vi "Project Manager.vi"() -> ()   [LabVIEW 2012]
doc: "This VI performs some project management operations on source trees. In particular, it is can be used to load VIs that are no subVI of the application such as instantiation templates, dynamically loaded VIs, test VIs and so on. By doing so, changes to subVIs or typedefs used throughout the source tree can be applied everywhere, evaluated (any VIs with broken arrows?), and reverted or saved as they are being made instead of waiting for any side effects to show the next time the using VIs in the source tree are loaded.\n\nTo deploy this VI, simply place it and its state typedef in the root directory of your projects VI source tree. To ease this migration, it is designed to not make use of any non-standard subVIs. When run, it will automatically list the VIs by recursing into the lower subdirectories. Thus, the collection of VIs being managed can be changed by moving the VI to a different source tree or by moving VIs into or outside the source tree."
uses:
  t_Project Manager States.ctl
panel:
  in  "exclude":string="^.*\\.ctt?$"
  in  "unload templates":bool
  in  "unload all":bool
  in  "include":string="^.*\\.[cv][ti][lt]?$"
  in  "directory/llb regexp":string
  in  "open selected":bool
  in  "reinitialize":bool
  in  "load all":bool
  in  "file list":i32[](listbox)
  in  "stop":bool
  in  "load selected":bool
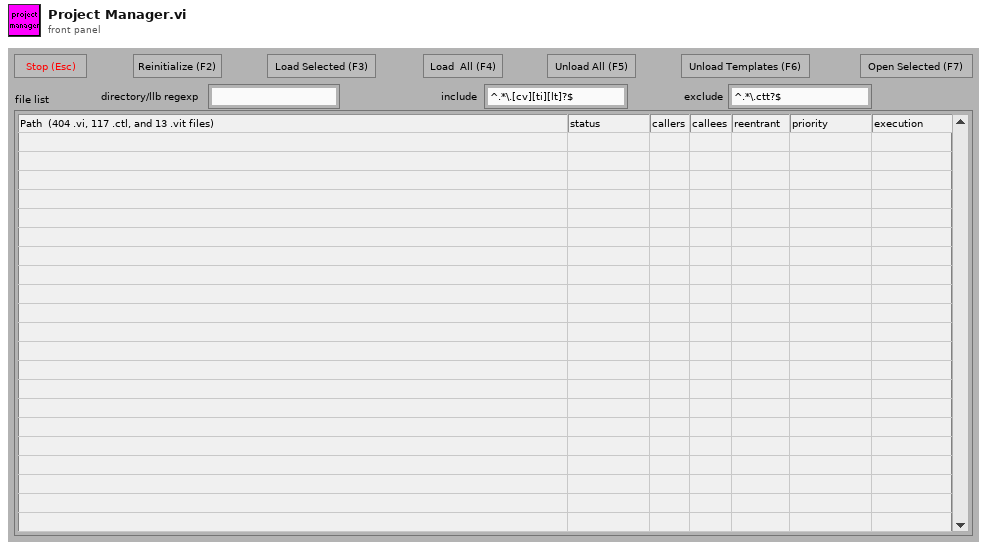
[diagram p1: front panel]
types:
  T1 = typedef "t_Project Manager States.ctl" = enum16{"empty queue", "adjust size", "load", "ld open", "ld calls", "ld system&exec", "unload", "unload templates", "open selected", "update stats", "ablement", "initialize", "cleanup", "stop"}
  T2 = enum32{"Bad", "Idle", "Run top level", "Running"}
  T3 = typedef "eventvkey.ctl" = enum16{"ASCII", "Enter", "Return", "Shift", "Ctrl", "Alt", "Cmd", "Opt", "Caps", "NumLock", "Clear", "Break", "Up", "Down", "Left", "Right", "Insert", "Delete", "Home", "End", "PageUp", "PageDown", "Escape", "Help", "Pause", "ScrollLock", "F1", "F2", "F3", "F4", "F5", "F6", "F7", "F8", "F9", "F10", "F11", "F12", "F13", "F14", "F15", "F16", "F17", "F18", "F19", "F20", "F21", "F22", "F23", "F24", "Play", "VolumeUp", "VolumeDown", "Mute", "Two Byte Char"}
  T4 = enum32{"invalid priority", "background priority", "normal priority", "above normal priority", "high priority", "time critical priority", "subroutine"}
  T5 = enum32{"invalid execution system", "user interface", "standard", "instrument i/o", "data acquisition", "other 1", "other 2", "same as caller"}
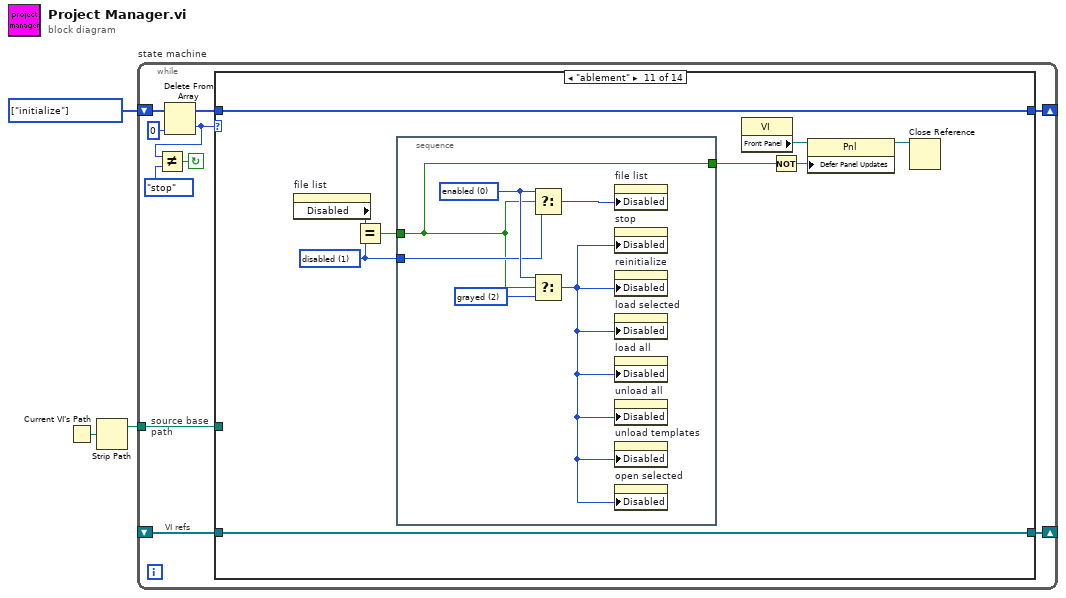
[diagram p0: block diagram]
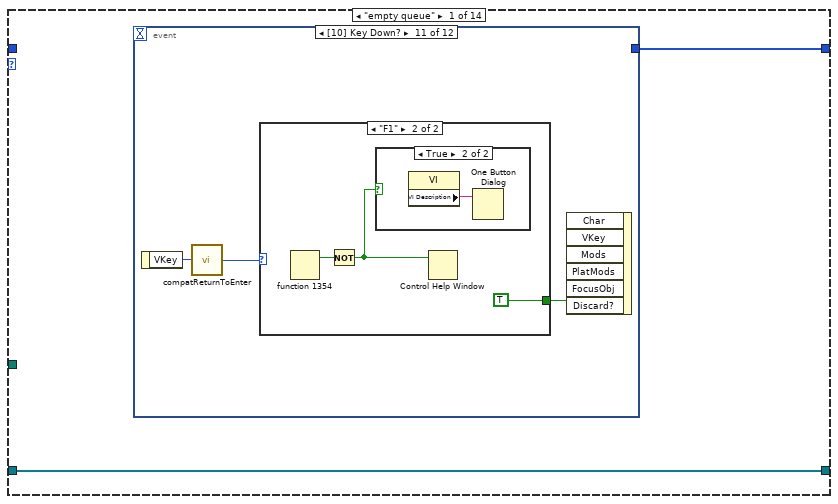
[diagram p2: hidden frame]
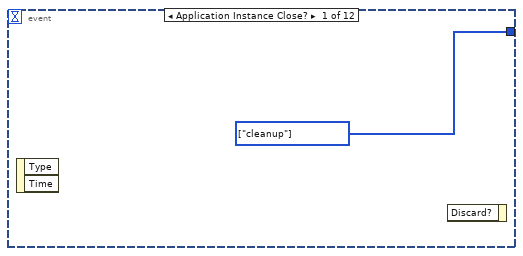
[diagram p3: hidden frame]
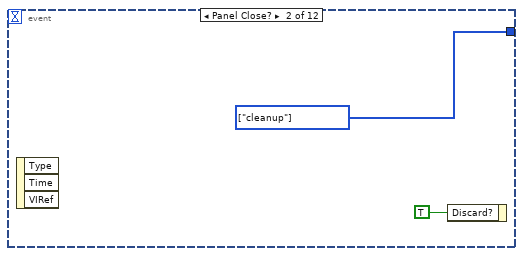
[diagram p4: hidden frame]
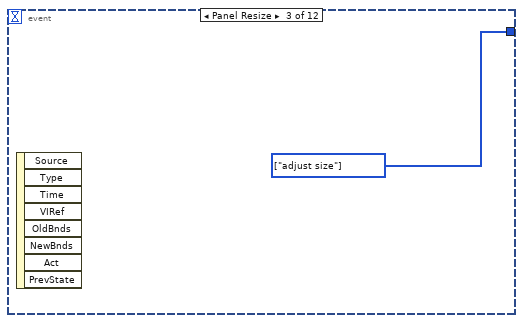
[diagram p5: hidden frame]
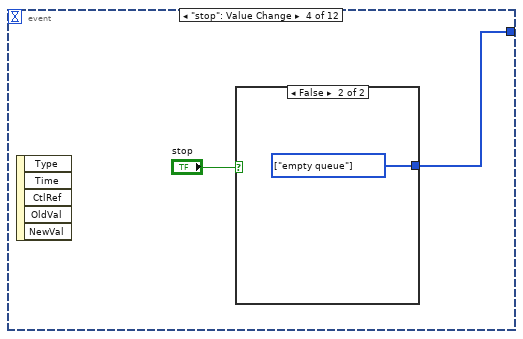
[diagram p6: hidden frame]
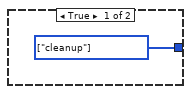
[diagram p7: hidden frame]
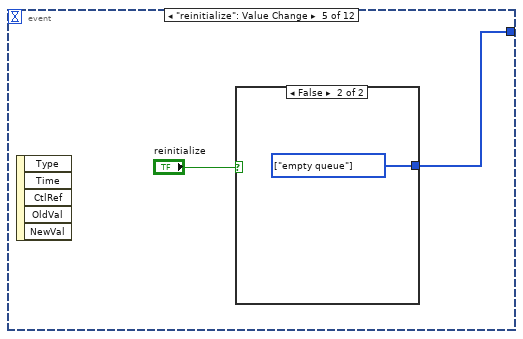
[diagram p8: hidden frame]
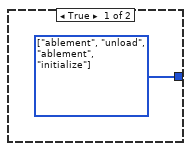
[diagram p9: hidden frame]
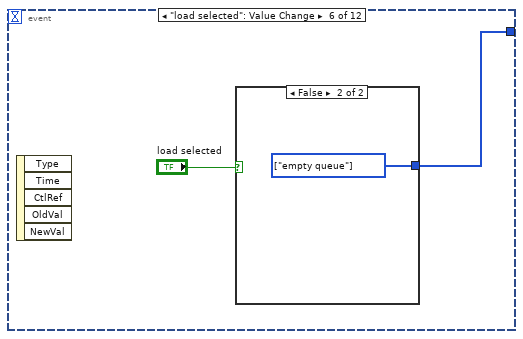
[diagram p10: hidden frame]
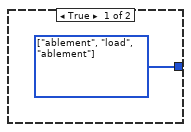
[diagram p11: hidden frame]
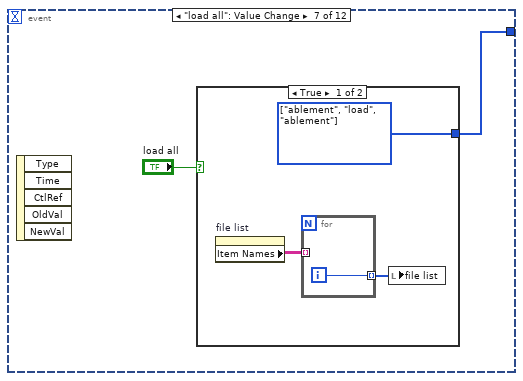
[diagram p12: hidden frame]
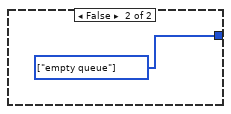
[diagram p13: hidden frame]
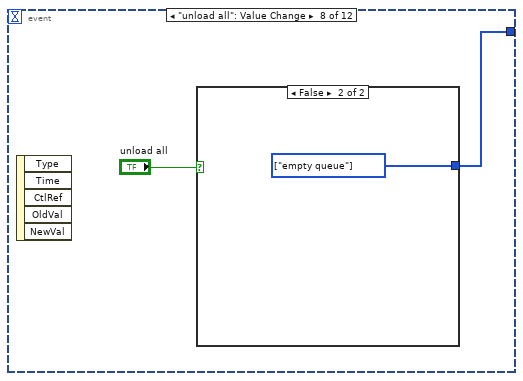
[diagram p14: hidden frame]
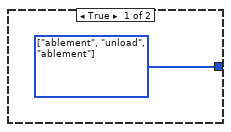
[diagram p15: hidden frame]
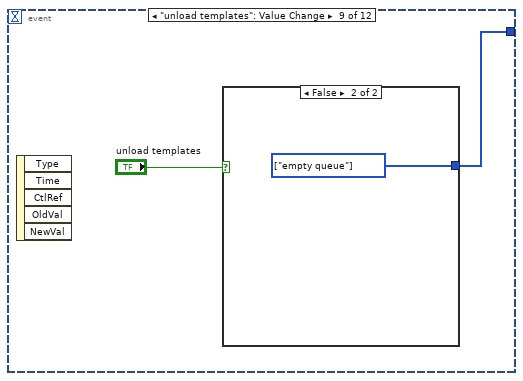
[diagram p16: hidden frame]
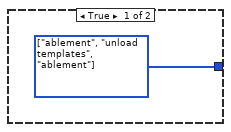
[diagram p17: hidden frame]
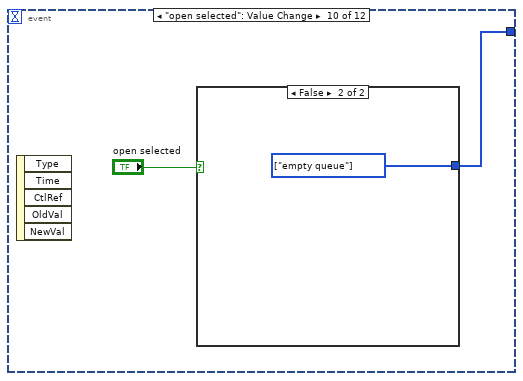
[diagram p18: hidden frame]
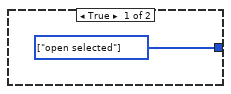
[diagram p19: hidden frame]
diagram:
  w3 = T1[] [enum."initialize"] items=["empty queue", "adjust size", "load", "ld open", "ld calls", "ld system&exec", "unload", "unload templates", "open selected", "update stats", "ablement", "initialize", "cleanup", "stop"] ("Array Constant")
  n1 = Current VI's Path() -> (path=w2:path)
  n2 = Strip Path(path=w2) -> (stripped path=w1:path)  [unwired: 1 out]
  n3 = while "state machine" {
    shift-left: w3 -> [w10]
    shift-right: [w13] -> _
    shift-right: [w5] -> _
    shift-left: _ -> [w6]
    tunnel: w1 -> [w4]
    stop <- w12 continue-if-true
    # "source base\npath"
    # "VI refs"
    n4 = Delete From Array(array=w10, index=0) -> (deleted portion=w8:T1, array with subset deleted=w9:T1[])  [unwired: 1 in]
    n5 = Not Equal?(x=w8, y=t_Project_Manager_States."stop" ("states")) -> (x != y?=w12:bool)
    n6 = case "Case" shown="\"ablement\"" w8 {
      tunnel: [w15 w63 w96 w130 w212 w285 w337 w359 w398 w432 w466 w492 w601 w603] -> w13
      tunnel: w9 -> [_ w63 w95 w130 w212 w285 w337 w359 w398 w432 w466 w497 _ w603]
      tunnel: w6 -> [w14 w62 w98 w129 w211 w284 w336 w358 w395 w431 w465 _ w598 w602]
      tunnel: [w14 w62 w98 w128 w211 w284 w335 w357 w395 w431 w465 w489 w598 w602] -> w5
      tunnel: w4 -> [_ _ _ w124 _ _ _ _ w394 _ _ w479 _ _]
      frame "empty queue" {
        n7 = event shown="[10] Key Down?" {
          selector: _ -> [_ _ _ _ _ _ _ _ _ _ _ _]
          dyn-events: _ -> [_ _ _ _ _ _ _ _ _ _ _ _]
          timeout: _ -> [_ _ _ _ _ _ _ _ _ _ _ _]
          tunnel: [w16 w18 w19 w21 w25 w28 w33 w40 w44 w48 _ _] -> w15
          event Application Instance Close? {
            w16 = T1[] [enum."cleanup"] items=["empty queue", "adjust size", "load", "ld open", "ld calls", "ld system&exec", "unload", "unload templates", "open selected", "update stats", "ablement", "initialize", "cleanup", "stop"] ("Array Constant")
            n8 = event-data() -> ()  [unwired: 1 in, 2 out]
            n9 = event-data() -> ()  [unwired: 2 in, 1 out]
          }
          event Panel Close? {
            w18 = T1[] [enum."cleanup"] items=["empty queue", "adjust size", "load", "ld open", "ld calls", "ld system&exec", "unload", "unload templates", "open selected", "update stats", "ablement", "initialize", "cleanup", "stop"] ("Array Constant")
            n10 = event-data() -> ()  [unwired: 1 in, 3 out]
            n11 = event-data("Discard?"=TRUE) -> ()  [unwired: 1 in, 1 out]
          }
          event Panel Resize {
            w19 = T1[] [enum."adjust size"] items=["empty queue", "adjust size", "load", "ld open", "ld calls", "ld system&exec", "unload", "unload templates", "open selected", "update stats", "ablement", "initialize", "cleanup", "stop"] ("Array Constant")
            n12 = event-data() -> ()  [unwired: 1 in, 8 out]
          }
          event "stop": Value Change {
            n13 = event-data() -> ()  [unwired: 1 in, 5 out]
            n14 = case shown="False" "stop" {
              tunnel: [w22 w23] -> w21
              frame True {
                w22 = T1[] [enum."cleanup"] items=["empty queue", "adjust size", "load", "ld open", "ld calls", "ld system&exec", "unload", "unload templates", "open selected", "update stats", "ablement", "initialize", "cleanup", "stop"] ("Array Constant")
              }
              frame False {
                w23 = T1[] [enum."empty queue"] items=["empty queue", "adjust size", "load", "ld open", "ld calls", "ld system&exec", "unload", "unload templates", "open selected", "update stats", "ablement", "initialize", "cleanup", "stop"] ("Array Constant")
              }
            }
          }
          event "reinitialize": Value Change {
            n15 = event-data() -> ()  [unwired: 1 in, 5 out]
            n16 = case shown="False" "reinitialize" {
              tunnel: [w26 w27] -> w25
              frame True {
                w26 = T1[] [enum."ablement", enum."unload", enum."ablement", enum."initialize"] items=["empty queue", "adjust size", "load", "ld open", "ld calls", "ld system&exec", "unload", "unload templates", "open selected", "update stats", "ablement", "initialize", "cleanup", "stop"] ("Array Constant")
              }
              frame False {
                w27 = T1[] [enum."empty queue"] items=["empty queue", "adjust size", "load", "ld open", "ld calls", "ld system&exec", "unload", "unload templates", "open selected", "update stats", "ablement", "initialize", "cleanup", "stop"] ("Array Constant")
              }
            }
          }
          event "load selected": Value Change {
            n17 = event-data() -> ()  [unwired: 1 in, 5 out]
            n18 = case shown="False" "load selected" {
              tunnel: [w30 w31] -> w28
              frame True {
                w30 = T1[] [enum."ablement", enum."load", enum."ablement"] items=["empty queue", "adjust size", "load", "ld open", "ld calls", "ld system&exec", "unload", "unload templates", "open selected", "update stats", "ablement", "initialize", "cleanup", "stop"] ("Array Constant")
              }
              frame False {
                w31 = T1[] [enum."empty queue"] items=["empty queue", "adjust size", "load", "ld open", "ld calls", "ld system&exec", "unload", "unload templates", "open selected", "update stats", "ablement", "initialize", "cleanup", "stop"] ("Array Constant")
              }
            }
          }
          event "load all": Value Change {
            n19 = event-data() -> ()  [unwired: 1 in, 5 out]
            n20 = case shown="True" "load all" {
              tunnel: [w34 w38] -> w33
              frame True {
                w34 = T1[] [enum."ablement", enum."load", enum."ablement"] items=["empty queue", "adjust size", "load", "ld open", "ld calls", "ld system&exec", "unload", "unload templates", "open selected", "update stats", "ablement", "initialize", "cleanup", "stop"] ("Array Constant")
                n21 = property on="file list" class="MCListbox (strict)"() -> ("Item Names"=w36:string[][])  [unwired: 2 in, 2 out]
                n22 = for {
                  tunnel: w36 -> [_] mode=indexing
                  tunnel: [w37] -> w35 mode=indexing
                  i -> [w37]
                }
                n23 = local write "file list"(w35) -> ()
              }
              frame False {
                w38 = T1[] [enum."empty queue"] items=["empty queue", "adjust size", "load", "ld open", "ld calls", "ld system&exec", "unload", "unload templates", "open selected", "update stats", "ablement", "initialize", "cleanup", "stop"] ("Array Constant")
              }
            }
          }
          event "unload all": Value Change {
            n24 = event-data() -> ()  [unwired: 1 in, 5 out]
            n25 = case shown="False" "unload all" {
              tunnel: [w41 w42] -> w40
              frame True {
                w41 = T1[] [enum."ablement", enum."unload", enum."ablement"] items=["empty queue", "adjust size", "load", "ld open", "ld calls", "ld system&exec", "unload", "unload templates", "open selected", "update stats", "ablement", "initialize", "cleanup", "stop"] ("Array Constant")
              }
              frame False {
                w42 = T1[] [enum."empty queue"] items=["empty queue", "adjust size", "load", "ld open", "ld calls", "ld system&exec", "unload", "unload templates", "open selected", "update stats", "ablement", "initialize", "cleanup", "stop"] ("Array Constant")
              }
            }
          }
          event "unload templates": Value Change {
            n26 = event-data() -> ()  [unwired: 1 in, 5 out]
            n27 = case shown="False" "unload templates" {
              tunnel: [w45 w46] -> w44
              frame True {
                w45 = T1[] [enum."ablement", enum."unload templates", enum."ablement"] items=["empty queue", "adjust size", "load", "ld open", "ld calls", "ld system&exec", "unload", "unload templates", "open selected", "update stats", "ablement", "initialize", "cleanup", "stop"] ("Array Constant")
              }
              frame False {
                w46 = T1[] [enum."empty queue"] items=["empty queue", "adjust size", "load", "ld open", "ld calls", "ld system&exec", "unload", "unload templates", "open selected", "update stats", "ablement", "initialize", "cleanup", "stop"] ("Array Constant")
              }
            }
          }
          event "open selected": Value Change {
            n28 = event-data() -> ()  [unwired: 1 in, 5 out]
            n29 = case shown="False" "open selected" {
              tunnel: [w49 w50] -> w48
              frame True {
                w49 = T1[] [enum."open selected"] items=["empty queue", "adjust size", "load", "ld open", "ld calls", "ld system&exec", "unload", "unload templates", "open selected", "update stats", "ablement", "initialize", "cleanup", "stop"] ("Array Constant")
              }
              frame False {
                w50 = T1[] [enum."empty queue"] items=["empty queue", "adjust size", "load", "ld open", "ld calls", "ld system&exec", "unload", "unload templates", "open selected", "update stats", "ablement", "initialize", "cleanup", "stop"] ("Array Constant")
              }
            }
          }
          event Key Down? {
            n30 = event-data() -> ("VKey"=w51:T3)  [unwired: 1 in]
            n31 = call <vilib>:"compatReturnToEnter.vi"("VKey"=w51) -> ("VKey"=w53:T3)
            n32 = case shown="\"F1\"" w53 {
              tunnel: [_ TRUE] -> w52
              frame Default {
              }
              frame "F1" {
                n33 = fn#1354() -> (1:w56:bool)  [unwired: 1 out]
                n34 = Not(x=w56) -> (.not. x?=w54:bool)
                n35 = case shown="True" w54 {
                  frame False {
                  }
                  frame True {
                    n36 = property class="VI"() -> ("VI Description"=w57:string)  [unwired: 2 in, 2 out]
                    n37 = One Button Dialog(message=w57) -> ()  [unwired: 1 in, 1 out]
                  }
                }
                n38 = Control Help Window(1:w54) -> ()  [unwired: 1 in]
              }
            }
            n39 = event-data("Discard?"=w52) -> ()  [unwired: 6 in, 1 out]
          }
          event event type 5.0.x8000000b {
            n40 = event-data() -> ("VKey"=w58:T3)  [unwired: 1 in, 9 out]
            n41 = call <vilib>:"compatReturnToEnter.vi"("VKey"=w58) -> ("VKey"=w60:T3)
            n42 = case shown="\"F1\"" w60 {
              tunnel: [_ TRUE] -> w59
              frame Default {
              }
              frame "F1" {
              }
            }
            n43 = event-data("Discard?"=w59) -> ()  [unwired: 6 in, 1 out]
          }
        }
      }
      frame "adjust size" {
        n44 = while {
          shift-right: [w69] -> _
          shift-left: _ -> [w66]
          shift-right: [w70] -> _
          shift-left: _ -> [w65]
          shift-right: [w67] -> _
          shift-left: _ -> [w71]
          shift-right: [w68] -> _
          shift-left: _ -> [w64]
          stop <- FALSE continue-if-true
          n45 = case shown="True" w71 {
            selector: w71 -> [_ w85]
            tunnel: [w74 w80] -> w70
            tunnel: [w76 w78] -> w69
            tunnel: [w74 w82] -> w68
            tunnel: [TRUE w85] -> w67
            tunnel: w66 -> [_ w79]
            tunnel: w65 -> [_ w81]
            tunnel: w64 -> [_ w83]
            frame False {
              n46 = property on="file list" class="MulticolumnListbox (strict)"("Active Cell:Active Cell"=cluster{i32, i32} {0, 0} ("Active Cell")) -> ("Bounds:Width"=w74:u32, "Active Cell:Cell Size:Width"=w76:u32)  [unwired: 2 in, 2 out]
            }
            frame True {
              n47 = property on="file list" class="MulticolumnListbox (strict)"() -> ("Bounds:Width"=w77:u32)  [unwired: 2 in, 2 out]
              n48 = Not Equal?(x=w77, y=w83) -> (x != y?=w84:bool)
              n49 = case shown="True" w84 {
                tunnel: [w88 w94] -> w82
                tunnel: w83 -> [w88 _]
                tunnel: w81 -> [w87 w91]
                tunnel: [w87 w91] -> w80
                tunnel: w79 -> [w86 w89]
                tunnel: [w86 w89] -> w78
                tunnel: w77 -> [_ w94]
                frame False {
                }
                frame True {
                  n50 = Subtract(x=w94, y=w91) -> (x-y=w93:u32)
                  n51 = Add(x=w93, y=w89) -> (x+y=w90:u32)
                  n52 = property on="file list" class="MulticolumnListbox (strict)"("Active Cell:Active Cell"=cluster{i32, i32} {-2, 0} ("Active Cell"), "Active Cell:Cell Size:Width"=w90) -> ()  [unwired: 2 in, 2 out]
                }
              }
            }
          }
        }
      }
      frame "load" {
        n53 = while "rebuild load list on first run or after load or recompile" {
          shift-left: _ -> [w101]
          shift-right: [w100] -> w97
          stop <- FALSE continue-if-true
          n54 = Array Size(array=w101) -> (size(s)=w102:i32)
          n55 = case shown="0" w102 {
            tunnel: [w103 w123] -> w100
            tunnel: w101 -> [w104 w123]
            frame 0 {
              n56 = while {
                shift-left: w104 -> [w113]
                shift-right: [w111] -> w103
                shift-left: _ -> [w115]
                shift-right: [w110] -> _
                i -> [w118]
                stop <- w106 continue-if-true
                n57 = To Unsigned Word Integer(number=w118) -> (unsigned 16bit integer=w116:u16)
                n58 = Type Cast(type=t_Project_Manager_States."initialize" ("states"), x=w116) -> (*(type *) &x=w112:T1)
                n59 = Format Into String(format string="%s" ("Format String"), w112) -> (resulting string=w110:string)  [unwired: 2 in, 1 out]
                n60 = Not Equal?(x=w110, y=w115) -> (x != y?=w106:bool)
                n61 = Match Pattern(string=w110, regular expression="^ld ") -> (offset past match=w108:i32)  [unwired: 1 in, 3 out]
                n62 = Greater Or Equal To 0?(x=w108) -> (x >= 0?=w107:bool)
                n63 = And(x=w107, y=w106) -> (x .and. y?=w105:bool)
                n64 = case shown="True" w105 {
                  tunnel: w113 -> [w119 w122]
                  tunnel: w112 -> [_ w121]
                  tunnel: [w119 w120] -> w111
                  frame False {
                  }
                  frame True {
                    n65 = Build Array (concatenate)(w122, w121) -> (w120:T1[])
                  }
                }
              }
            }
            frame Default {
            }
          }
        }
        n66 = Build Array (concatenate)(w97, w95) -> (w96:T1[])
      }
      frame "ld open" {
        n67 = property on="file list" class="MCListbox (strict)"() -> ("Item Names"=w127:string[][])  [unwired: 2 in, 2 out]
        n68 = Array Size(array="file list") -> (size(s)=w126:i32)
        n69 = case shown="Default" w126 {
          tunnel: "file list" -> [_ w137]
          tunnel: w127 -> [_ w136]
          tunnel: w129 -> [w131 w135]
          tunnel: [w131 w134] -> w128
          tunnel: w124 -> [_ w132]
          frame 0 {
          }
          frame Default {
            n70 = while {
              shift-right: [w147] -> _
              shift-left: w137 -> [w149]
              shift-right: [w143] -> w133
              shift-left: w136 -> [w148]
              shift-right: [w144] -> w134
              shift-left: w135 -> [w142]
              tunnel: w132 -> [w138]
              stop <- w145 stop-if-true
              n71 = Delete From Array(array=w149, index=0) -> (deleted portion=w141:i32, array with subset deleted=w147:i32[])  [unwired: 1 in]
              n72 = Index Array(array=w142, index=w141) -> (element=w140:refnum<vi>)
              n73 = Not A Number/Path/Refnum?(number/path/refnum=w140) -> (NaN/Path/Refnum?=w139:bool)
              n74 = case "not loaded yet?" shown="True" w139 {
                tunnel: w148 -> [w152 w170]
                tunnel: w142 -> [w151 w169]
                tunnel: [w151 w168] -> w144
                tunnel: [w152 w157] -> w143
                tunnel: w141 -> [_ w156]
                tunnel: w138 -> [_ w155]
                frame False {
                }
                frame True {
                  # "template?"
                  n75 = Index Array(array=w170, index (row)=w156, index (col)=0 ("disabled index (col)")) -> (element=w159:string)
                  n76 = String To Path(string=w159) -> (path=w154:path)
                  n77 = Match Pattern(string=w159, regular expression="\\.[vV][iI][tT}$") -> (offset past match=w163:i32)  [unwired: 1 in, 3 out]
                  n78 = Greater Or Equal To 0?(x=w163) -> (x >= 0?=w161:bool)
                  n79 = Build Path(base path=w155, name or relative path=w154) -> (appended path=w153:path)
                  n80 = Select(t=2 ("options"), s=w161, f=0 ("options")) -> (s? t:f=w158:i32)
                  n81 = Open VI Reference(vi path=w153, options=w158) -> (vi reference=w172:refnum<vi>, error out=w173:errorcluster)  [unwired: 4 in]
                  n82 = case shown="No Error" w173 {
                    tunnel: w172 -> [w177 _]
                    tunnel: [w181 "Load error"] -> w171
                    tunnel: w169 -> [w180 w204]
                    tunnel: [w179 w203] -> w168
                    tunnel: [w178 u32 16727100] -> w167
                    tunnel: w156 -> [w176 w202]
                    frame No Error {
                      n83 = stacked-sequence {
                        tunnel: [w188 _] -> w181
                        tunnel: w180 -> [w186 _]
                        tunnel: [w185 _] -> w179
                        tunnel: [w184 _] -> w178
                        tunnel: w177 -> [w183 w198]
                        tunnel: w176 -> [w182 _]
                        frame #0 {
                          n84 = property class="VI"(reference=w183) -> (error out=w187:errorcluster, "Execution:State"=w190:T2)  [unwired: 1 in, 1 out]
                          n85 = Equal?(x=w190, y=T2."Bad" ("Execution:State")) -> (x = y?=w189:bool)
                          n86 = case shown="True" w189 {
                            tunnel: ["Loaded" "Broken"] -> w188
                            tunnel: w187 -> [_ _]
                            tunnel: [u32 15790320 u32 16727100] -> w184
                            frame False {
                            }
                            frame True {
                            }
                          }
                          n87 = Replace Array Subset(array=w186, new element=w183, index=w182) -> (w185:refnum<vi>[])
                        }
                        frame #1 {
                          # "we don't want to have front\npanels set to show on load\npop open"
                          n88 = property class="VI"(reference=w198) -> (reference out=w197:refnum<vi>, "Execution:Show Front Panel On Load"=w196:bool)  [unwired: 1 in, 1 out]
                          n89 = case shown="True" w196 {
                            tunnel: w197 -> [_ w200]
                            frame False {
                            }
                            frame True {
                              n90 = property class="VI"(reference=w200, "Front Panel Window:Open"=FALSE) -> ()  [unwired: 1 in, 2 out]
                            }
                          }
                        }
                      }
                    }
                    frame Error {
                      n91 = Replace Array Subset(array=w204, new element=refnum<k0> refnum, index=w202) -> (w203:refnum<vi>[])
                    }
                  }
                  n92 = Bundle(w156, "element"=1) -> (w166:cluster{i32, "element":i32})  [unwired: 1 in]
                  n93 = property on="file list" class="MCListbox (strict)"("Active Cell:Active Cell"=w166, "Active Cell:Cell Background Color"=w167) -> ()  [unwired: 2 in, 2 out]
                  n94 = Replace Array Subset(array=w170, new element=w171, index (row)=w156, index (col)=1 ("disabled index (col)")) -> (w157:string[][])
                }
              }
              n95 = Array Size(array=w147) -> (size(s)=w146:i32)
              n96 = local write "file list"(w147) -> ()
              n97 = Equal To 0?(x=w146) -> (x = 0?=w145:bool)
            }
            n98 = property on="file list" class="MCListbox (strict)"("Item Names"=w133) -> ()  [unwired: 2 in, 2 out]
          }
        }
      }
      frame "ld calls" {
        w207 = TRUE
        # "stop LV8\nfrom\ncomplaining"
        n99 = property on="file list" class="MCListbox (strict)"() -> ("Item Names"=w210:string[][])  [unwired: 2 in, 2 out]
        n100 = And(x=w207, y=w207) -> (x .and. y?=w208:bool)
        n101 = for {
          tunnel: w211 -> [w223] mode=indexing
          shift-right: [w218] -> w209
          shift-left: w210 -> [w216]
          tunnel: w208 -> [w213]
          i -> [w215]
          n102 = Not A Number/Path/Refnum?(number/path/refnum=w223) -> (NaN/Path/Refnum?=w224:bool)
          n103 = case shown="False" w224 {
            tunnel: w223 -> [w244 _]
            tunnel: [w240 w281] -> w219
            tunnel: [w239 w281] -> w220
            tunnel: [w232 w280] -> w217
            tunnel: w216 -> [w238 w280]
            tunnel: w215 -> [w236 w279]
            tunnel: [w236 w279] -> w214
            tunnel: w213 -> [w225 _]
            frame False {
              # "Mark stuff that should\nbe called but isn't or\nshould not be used\nmultiple times."
              n104 = property class="VI"(reference=w244) -> ("Callers' Names"=w243:string[], "Callees' Names"=w242:string[])  [unwired: 1 in, 2 out]
              n105 = Array Size(array=w243) -> (size(s)=w235:i32)
              n106 = Array Size(array=w242) -> (size(s)=w241:i32)
              n107 = Equal To 0?(x=w235) -> (x = 0?=w237:bool)
              n108 = Greater?(x=w235, y=1) -> (0:w233:bool)
              n109 = case shown="True" w225 {
                tunnel: w238 -> [w245 w251]
                tunnel: w237 -> [w246 w263]
                tunnel: w236 -> [_ w262]
                tunnel: [w246 w258] -> w229
                tunnel: w233 -> [_ w256]
                tunnel: [w245 w251] -> w232
                frame False {
                }
                frame True {
                  n110 = Index Array(array=w251, index (row)=w262, index (col)=0 ("disabled index (col)")) -> (element=w259:string)
                  n111 = To Lower Case(string=w259) -> (all lower case string=w248:string)
                  n112 = Match Pattern(string=w248, regular expression="states\\.") -> (offset past match=w261:i32)  [unwired: 1 in, 3 out]
                  n113 = Match Pattern(string=w248, regular expression="\\.ctl$") -> (offset past match=w275:i32)  [unwired: 1 in, 3 out]
                  n114 = Match Pattern(string=w248, regular expression="\\.vi$") -> (offset past match=w272:i32)  [unwired: 1 in, 3 out]
                  n115 = Match Pattern(string=w248, regular expression="subvis") -> (offset past match=w271:i32)  [unwired: 1 in, 3 out]
                  n116 = Match Pattern(string=w248, regular expression="objects") -> (offset past match=w270:i32)  [unwired: 1 in, 3 out]
                  n117 = Match Pattern(string=w248, regular expression="library") -> (offset past match=w250:i32)  [unwired: 1 in, 3 out]
                  n118 = Greater Or Equal To 0?(x=w261) -> (x >= 0?=w252:bool)
                  n119 = Greater Or Equal To 0?(x=w275) -> (x >= 0?=w254:bool)
                  n120 = Greater Or Equal To 0?(x=w272) -> (x >= 0?=w267:bool)
                  n121 = Greater Or Equal To 0?(x=w271) -> (x >= 0?=w269:bool)
                  n122 = Greater Or Equal To 0?(x=w270) -> (x >= 0?=w268:bool)
                  n123 = Greater Or Equal To 0?(x=w250) -> (x >= 0?=w247:bool)
                  n124 = Compound Arithmetic op=OR(w269, w268, w247) -> (w266:bool)
                  n125 = And(x=w267, y=w266) -> (x .and. y?=w265:bool)
                  n126 = And(x=w252, y=w254) -> (x .and. y?=w253:bool)
                  n127 = Or(x=w254, y=w265) -> (x .or. y?=w264:bool)
                  n128 = And(x=w263, y=w264) -> (x .and. y?=w257:bool)
                  n129 = And(x=w256, y=w253) -> (x .and. y?=w255:bool)
                  n130 = Or(x=w255, y=w257) -> (x .or. y?=w258:bool)
                }
              }
              n131 = Select(t=u32 16752680, s=w229, f=u32 15790320) -> (s? t:f=w226:u32)
              n132 = Bundle(w236, "element"=2) -> (w231:cluster{i32, "element":i32})  [unwired: 1 in]
              n133 = Format Into String(w235) -> (resulting string=w239:string)  [unwired: 3 in, 1 out]
              n134 = Format Into String(w241) -> (resulting string=w240:string)  [unwired: 3 in, 1 out]
              n135 = property on="file list" class="MCListbox (strict)"("Active Cell:Active Cell"=w231, "Active Cell:Cell Background Color"=w226) -> ()  [unwired: 2 in, 2 out]
            }
            frame True {
              w281 = ""
            }
          }
          n136 = Replace Array Subset(array=w217, new element #1=w220, index (row) #1=w214, index (col) #1=2 ("disabled index (col)"), new element #2=w219, index (row) #2=w214, index (col) #2=3 ("disabled index (col)")) -> (w218:string[][])
        }
        n137 = property on="file list" class="MCListbox (strict)"("Item Names"=w209) -> ()  [unwired: 2 in, 2 out]
      }
      frame "ld system&exec" {
        n138 = property on="file list" class="MCListbox (strict)"() -> ("Item Names"=w283:string[][])  [unwired: 2 in, 2 out]
        n139 = for {
          tunnel: w284 -> [w298] mode=indexing
          shift-right: [w299] -> w282
          shift-left: w283 -> [w301]
          i -> [w287]
          # "VIs prefixed with \"re_\" that are not reentrant are flagged.\nReentrant VIs tend to be made non-reentrant every now\nand then so as to allow debugging. This facility allows you\nto easily spot those VIs that should be reset to reentrant."
          n140 = Not A Number/Path/Refnum?(number/path/refnum=w298) -> (NaN/Path/Refnum?=w302:bool)
          n141 = case shown="False" w302 {
            tunnel: w298 -> [w323 _]
            tunnel: [w315 w329] -> w291
            tunnel: [w316 w328] -> w295
            tunnel: [w305 w329] -> w292
            tunnel: [w308 w329] -> w290
            tunnel: [w311 w328] -> w286
            frame False {
              n142 = property class="VI"(reference=w323) -> ("Is System VI"=w312:bool, "Execution:Priority"=w309:T4, "Execution:Preferred Exec System"=w307:T5, "Execution:Is Reentrant"=w306:bool, "VI Name"=w322:string)  [unwired: 1 in, 2 out]
              n143 = Match Pattern(string=w322, regular expression="^[rR][eE]_") -> (offset past match=w320:i32)  [unwired: 1 in, 3 out]
              n144 = Greater Or Equal To 0?(x=w320) -> (x >= 0?=w319:bool)
              n145 = Not Equal?(x=w306, y=w319) -> (x != y?=w318:bool)
              n146 = case shown="Default" w309 {
                selector: w309 -> [_ w326]
                tunnel: [_ w327] -> w315
                frame "invalid priority" {
                }
                frame Default {
                  n147 = Format Into String(w326) -> (resulting string=w327:string)  [unwired: 3 in, 1 out]
                }
              }
              n148 = case shown="Default" w307 {
                selector: w307 -> [_ w324]
                tunnel: [_ w325] -> w308
                frame "invalid execution system" {
                }
                frame Default {
                  n149 = Format Into String(w324) -> (resulting string=w325:string)  [unwired: 3 in, 1 out]
                }
              }
              n150 = Select(t="true", s=w306, f="") -> (s? t:f=w305:string)
              n151 = Select(t=u32 13816530, s=w312, f=u32 15790320) -> (s? t:f=w311:u32)
              n152 = Select(t=u32 16752680, s=w318, f=u32 15790320) -> (s? t:f=w316:u32)
            }
            frame True {
              w328 = u32 15790320
              w329 = ""
            }
          }
          n153 = Bundle(w287, "element"=4) -> (w297:cluster{i32, "element":i32})  [unwired: 1 in]
          n154 = Bundle(w287, "element"=0) -> (w288:cluster{i32, "element":i32})  [unwired: 1 in]
          n155 = property on="file list" class="MCListbox (strict)"("Active Cell:Active Cell"=w297, "Active Cell:Cell Background Color"=w295, "Active Cell:Active Cell"=w288, "Active Cell:Cell Background Color"=w286) -> ()  [unwired: 2 in, 2 out]
          n156 = Replace Array Subset(array=w301, new element #1=w292, index (row) #1=w287, index (col) #1=4 ("disabled index (col)"), new element #2=w291, index (row) #2=w287, index (col) #2=5 ("disabled index (col)"), new element #3=w290, index (row) #3=w287, index (col) #3=6 ("disabled index (col)")) -> (w299:string[][])
        }
        n157 = property on="file list" class="MCListbox (strict)"("Item Names"=w282) -> ()  [unwired: 2 in, 2 out]
      }
      frame "unload" {
        w331 = -2 ("element")
        n158 = property on="file list" class="MCListbox (strict)"() -> ("Item Names"=w334:string[][])  [unwired: 2 in, 2 out]
        n159 = for {
          tunnel: w336 -> [w346] mode=indexing
          tunnel: [refnum<vi> refnum ("vi reference")] -> w335 mode=indexing
          shift-right: [w342] -> w333
          shift-left: w334 -> [w343]
          i -> [w339]
          n160 = Array Size(array=w343) -> (size(s)=w345:i32[])
          n161 = Not A Number/Path/Refnum?(number/path/refnum=w346) -> (NaN/Path/Refnum?=w347:bool)
          n162 = case shown="False" w347 {
            tunnel: w346 -> [w354 _]
            frame False {
              n163 = Close Reference(reference=w354) -> ()  [unwired: 1 in, 1 out]
            }
            frame True {
            }
          }
          n164 = Index Array(array=w345, index=1) -> (element=w341:i32)
          n165 = Decrement(x=w341) -> (x-1=w340:i32)
          n166 = for {
            N: w340 -> [_]
            tunnel: w339 -> [w353]
            shift-right: [w348] -> w342
            shift-left: w343 -> [w352]
            i -> [w351]
            n167 = Increment(x=w351) -> (x+1=w350:i32)
            n168 = Replace Array Subset(array=w352, new element="", index (row)=w353, index (col)=w350) -> (w348:string[][])
          }
        }
        n169 = Bundle("element"=w331, "element"=w331) -> (w332:cluster{"element":i32, "element":i32})  [unwired: 1 in]
        n170 = property on="file list" class="MCListbox (strict)"("Item Names"=w333, "Active Cell:Active Cell"=w332, "Active Cell:Cell Background Color"=u32 15790320) -> ()  [unwired: 2 in, 2 out]
      }
      frame "unload templates" {
        n171 = property on="file list" class="MCListbox (strict)"() -> ("Item Names"=w356:string[][])  [unwired: 2 in, 2 out]
        n172 = for {
          tunnel: w358 -> [w368] mode=indexing
          tunnel: [w369] -> w357 mode=indexing
          shift-right: [w367] -> w355
          shift-left: w356 -> [w362]
          i -> [w361]
          n173 = Index Array(array=w362, index (row)=w361, index (col)=0 ("disabled index (col)")) -> (element=w363:string)
          n174 = Match Pattern(string=w363, regular expression="\\.[vV][iI][tT}$") -> (offset past match=w364:i32)  [unwired: 1 in, 3 out]
          n175 = Greater Or Equal To 0?(x=w364) -> (x >= 0?=w360:bool)
          n176 = case shown="True" w360 {
            tunnel: [w371 refnum<vi> refnum ("vi reference")] -> w369
            tunnel: w368 -> [w371 w385]
            tunnel: w362 -> [w370 w382]
            tunnel: [w370 w381] -> w367
            tunnel: w361 -> [_ w374]
            frame False {
            }
            frame True {
              w372 = u32 15790320
              n177 = Array Size(array=w382) -> (size(s)=w384:i32[])
              n178 = Not A Number/Path/Refnum?(number/path/refnum=w385) -> (NaN/Path/Refnum?=w386:bool)
              n179 = case shown="False" w386 {
                tunnel: w385 -> [w393 _]
                frame False {
                  n180 = Close Reference(reference=w393) -> ()  [unwired: 1 in, 1 out]
                }
                frame True {
                }
              }
              n181 = Index Array(array=w384, index=1) -> (element=w380:i32)
              n182 = Bundle(w374, "element"=1) -> (w378:cluster{i32, "element":i32})  [unwired: 1 in]
              n183 = Bundle(w374, "element"=4) -> (w376:cluster{i32, "element":i32})  [unwired: 1 in]
              n184 = Decrement(x=w380) -> (x-1=w379:i32)
              n185 = for {
                N: w379 -> [_]
                tunnel: w374 -> [w392]
                shift-right: [w387] -> w381
                shift-left: w382 -> [w391]
                i -> [w390]
                n186 = Increment(x=w390) -> (x+1=w389:i32)
                n187 = Replace Array Subset(array=w391, new element="", index (row)=w392, index (col)=w389) -> (w387:string[][])
              }
              n188 = property on="file list" class="MCListbox (strict)"("Active Cell:Active Cell"=w378, "Active Cell:Cell Background Color"=w372, "Active Cell:Active Cell"=w376, "Active Cell:Cell Background Color"=w372) -> ()  [unwired: 2 in, 2 out]
            }
          }
        }
        n189 = property on="file list" class="MCListbox (strict)"("Item Names"=w355) -> ()  [unwired: 2 in, 2 out]
      }
      frame "open selected" {
        n190 = property on="file list" class="MCListbox (strict)"() -> ("Item Names"=w397:string[][])  [unwired: 2 in, 2 out]
        n191 = local read "file list"() -> (w396:i32[])
        n192 = for {
          tunnel: w397 -> [w414]
          tunnel: w396 -> [w410] mode=indexing
          tunnel: w394 -> [w399]
          # "template?"
          n193 = Index Array(array=w414, index (row)=w410, index (col)=0 ("disabled index (col)")) -> (element=w409:string)
          n194 = Match Pattern(string=w409, regular expression="\\.[vV][iI][tT}$") -> (offset past match=w407:i32)  [unwired: 1 in, 3 out]
          n195 = String To Path(string=w409) -> (path=w400:path)
          n196 = Greater Or Equal To 0?(x=w407) -> (x >= 0?=w405:bool)
          n197 = Build Path(base path=w399, name or relative path=w400) -> (appended path=w401:path)
          n198 = Select(t=2 ("options"), s=w405, f=0 ("options")) -> (s? t:f=w403:i32)
          n199 = Open VI Reference(vi path=w401, options=w403) -> (vi reference=w415:refnum<vi>, error out=w413:errorcluster)  [unwired: 4 in]
          n200 = property class="VI"(reference=w415, error in=w413, "Front Panel Window:Open"=TRUE, "Front Panel Window:Is Frontmost"=TRUE) -> (reference out=w411:refnum<vi>)  [unwired: 1 out]
          n201 = Close Reference(reference=w411) -> ()  [unwired: 1 in, 1 out]
        }
      }
      frame "update stats" {
        n202 = property on="file list" class="MCListbox (strict)"() -> ("Column Header Strings[]"=w424:string[], "Item Names"=w430:string[][])  [unwired: 2 in, 2 out]
        n203 = Index Array(array=w430, index (col)=0 ("disabled index (col)")) -> (element=w428:string[])  [unwired: 1 in]
        n204 = for {
          tunnel: w428 -> [w442] mode=indexing
          shift-right: [w437] -> w421
          shift-left: 0 ("disabled index (col)") -> [w438]
          shift-right: [w436] -> w420
          shift-left: 0 ("disabled index (col)") -> [w435]
          shift-right: [w434] -> w419
          shift-left: 0 ("disabled index (col)") -> [w433]
          n205 = To Lower Case(string=w442) -> (all lower case string=w440:string)
          n206 = Match Pattern(string=w440, regular expression="\\.[~\\.]+$") -> (match substring=w439:string)  [unwired: 1 in, 3 out]
          n207 = case shown="Default" w439 {
            tunnel: [w445 w446 w453 w457] -> w437
            tunnel: w438 -> [w445 w449 w453 w457]
            tunnel: w435 -> [w444 w448 w452 w456]
            tunnel: [w444 w448 w450 w456] -> w436
            tunnel: [w443 w447 w451 w454] -> w434
            tunnel: w433 -> [w443 w447 w451 w455]
            frame Default {
            }
            frame ".vi" {
              n208 = Increment(x=w449) -> (x+1=w446:i32)
            }
            frame ".ctl" {
              n209 = Increment(x=w452) -> (x+1=w450:i32)
            }
            frame ".vit" {
              n210 = Increment(x=w455) -> (x+1=w454:i32)
            }
          }
        }
        n211 = Format Into String(format string="Path  (%d .vi, %d .ctl, and %d .vit files)", w421, w420, w419) -> (resulting string=w417:string)  [unwired: 2 in, 1 out]
        n212 = Replace Array Subset(array=w424, new element=w417, index=0) -> (w422:string[])
        n213 = property on="file list" class="MCListbox (strict)"("Column Header Strings[]"=w422) -> ()  [unwired: 2 in, 2 out]
      }
      frame "ablement" {
        w460 = u8 1 items=["enabled", "disabled", "grayed"] ("disabled state")
        n214 = property on="file list" class="MCListbox (strict)"() -> ("Disabled"=w464:u8)  [unwired: 2 in, 2 out]
        n215 = Equal?(x=w464, y=w460) -> (x = y?=w459:bool)
        n216 = stacked-sequence {
          tunnel: w460 -> [w469]
          tunnel: w459 -> [w468]
          tunnel: [w468] -> w458
          frame #0 {
            w471 = u8 2 items=["enabled", "disabled", "grayed"] ("disabled state")
            w470 = u8 0 items=["enabled", "disabled", "grayed"] ("disabled state")
            n217 = Select(t=w470, s=w468, f=w469) -> (s? t:f=w472:u8)
            n218 = Select(t=w470, s=w468, f=w471) -> (s? t:f=w467:u8)
            n219 = property on="file list" class="MCListbox (strict)"("Disabled"=w472) -> ()  [unwired: 2 in, 2 out]
            n220 = property on="stop" class="Bool"("Disabled"=w467) -> ()  [unwired: 2 in, 2 out]
            n221 = property on="reinitialize" class="Bool"("Disabled"=w467) -> ()  [unwired: 2 in, 2 out]
            n222 = property on="load selected" class="Bool"("Disabled"=w467) -> ()  [unwired: 2 in, 2 out]
            n223 = property on="load all" class="Bool"("Disabled"=w467) -> ()  [unwired: 2 in, 2 out]
            n224 = property on="unload all" class="Bool"("Disabled"=w467) -> ()  [unwired: 2 in, 2 out]
            n225 = property on="unload templates" class="Bool"("Disabled"=w467) -> ()  [unwired: 2 in, 2 out]
            n226 = property on="open selected" class="Bool"("Disabled"=w467) -> ()  [unwired: 2 in, 2 out]
          }
        }
        n227 = property class="VI"() -> ("Front Panel"=w463:refnum<vi>)  [unwired: 2 in, 2 out]
        n228 = Not(x=w458) -> (.not. x?=w462:bool)
        n229 = property class="Pnl"(reference=w463, "Defer Panel Updates"=w462) -> (reference out=w461:refnum<vi>)  [unwired: 1 in, 1 out]
        n230 = Close Reference(reference=w461) -> ()  [unwired: 1 in, 1 out]
      }
      frame "initialize" {
        w482 = T1[] [enum."update stats", enum."adjust size", enum."ablement"] items=["empty queue", "adjust size", "load", "ld open", "ld calls", "ld system&exec", "unload", "unload templates", "open selected", "update stats", "ablement", "initialize", "cleanup", "stop"] ("Array Constant")
        w486 = u8 1 items=["enabled", "disabled", "grayed"] ("disabled state")
        w494 = 0 ("dimension size")
        # "avoid LV7 bug"
        n231 = Path To String(path=w479) -> (string=w478:string)
        n232 = String Length(string=w478) -> (length=w477:i32)
        n233 = local write "file list"(i32[] [] ("unit tests")) -> ()
        n234 = Initialize Array("", w494, w494) -> (w495:string[][])
        n235 = Increment(x=w477) -> (x+1=w476:i32)
        n236 = Build Array(w479) -> (w485:path[])
        n237 = while "recursively list directories & llbs" {
          shift-left: errorcluster {"status"=FALSE, "code"=0, "source"=""} ("error IO") -> [w516]
          shift-right: [w507] -> w484
          shift-left: w485 -> [w512]
          shift-right: [w511] -> w475
          i -> [w510]
          stop <- w504 stop-if-true
          n238 = Index Array(array=w512, index=w510) -> (element=w514:path)
          n239 = List Folder(path=w514, error in=w516) -> (filenames=w503:string[], folder names=w515:string[], error out=w513:errorcluster)  [unwired: 2 in, 1 out]
          n240 = case shown="No Error" w513 {
            selector: w513 -> [w522 w541]
            tunnel: w515 -> [w521 _]
            tunnel: w514 -> [w519 _]
            tunnel: w512 -> [w524 w542]
            tunnel: [w523 w542] -> w511
            tunnel: [w522 w541] -> w507
            tunnel: w503 -> [w517 _]
            frame No Error {
              n241 = for {
                tunnel: w521 -> [w539] mode=indexing
                tunnel: w519 -> [w540]
                tunnel: [w538] -> w520 mode=indexing
                n242 = Build Path(base path=w540, name or relative path=w539) -> (appended path=w538:path)
              }
              n243 = for {
                tunnel: w519 -> [w531]
                tunnel: w517 -> [w528] mode=indexing
                shift-right: [w529] -> w518
                shift-left: w520 -> [w530]
                n244 = Match Pattern(string=w528, regular expression=".\\.[lL][lL][bB]$") -> (offset past match=w526:i32)  [unwired: 1 in, 3 out]
                n245 = Greater Or Equal To 0?(x=w526) -> (x >= 0?=w525:bool)
                n246 = case shown="True" w525 {
                  tunnel: w531 -> [_ w537]
                  tunnel: w530 -> [w532 w534]
                  tunnel: [w532 w536] -> w529
                  tunnel: w528 -> [_ w533]
                  frame False {
                  }
                  frame True {
                    n247 = Build Path(base path=w537, name or relative path=w533) -> (appended path=w535:path)
                    n248 = Build Array (concatenate)(w534, w535) -> (w536:path[])
                  }
                }
              }
              n249 = Build Array (concatenate)(w524, w518) -> (w523:path[])
            }
            frame Error {
            }
          }
          n250 = Array Size(array=w511) -> (size(s)=w509:i32)
          n251 = Increment(x=w510) -> (x+1=w508:i32)
          n252 = Less Or Equal?(x=w509, y=w508) -> (x <= y?=w506:bool)
          n253 = Unbundle By Name(w507) -> ("status"=w505:bool)
          n254 = Or(x=w505, y=w506) -> (x .or. y?=w504:bool)
        }
        n255 = Sort 1D Array(array=w475) -> (sorted array=w474:path[])
        n256 = Sort 1D Array(array=w474) -> (sorted array=w473:path[])
        n257 = for "list all matching files in matching directories/llbs" {
          tunnel: w473 -> [w550] mode=indexing
          shift-right: [w553] -> w481
          shift-left: w484 -> [w554]
          shift-right: [w551] -> w491
          shift-left: w495 -> [w552]
          tunnel: w476 -> [w543]
          n258 = Path To String(path=w550) -> (string=w549:string)
          n259 = To Lower Case(string=w549) -> (all lower case string=w548:string)
          n260 = To Lower Case(string="directory/llb regexp") -> (all lower case string=w545:string)
          n261 = Match Pattern(string=w548, regular expression=w545) -> (offset past match=w547:i32)  [unwired: 1 in, 3 out]
          n262 = Greater Or Equal To 0?(x=w547) -> (x >= 0?=w546:bool)
          n263 = case shown="True" w546 {
            tunnel: w550 -> [_ w567]
            tunnel: w554 -> [w556 w566]
            tunnel: [w556 w561] -> w553
            tunnel: w552 -> [w555 w562]
            tunnel: [w555 w560] -> w551
            tunnel: w543 -> [_ w557]
            frame False {
            }
            frame True {
              n264 = List Folder(path=w567, error in=w566) -> (path out=w564:path, filenames=w563:string[], error out=w565:errorcluster)  [unwired: 2 in, 1 out]
              n265 = for {
                shift-right: [w580] -> w561
                shift-left: w565 -> [w581]
                tunnel: w564 -> [w584]
                tunnel: w563 -> [w576] mode=indexing
                shift-right: [w582] -> w560
                shift-left: w562 -> [w583]
                tunnel: "include" -> [w577]
                tunnel: "exclude" -> [w573]
                tunnel: w557 -> [w568]
                n266 = To Lower Case(string=w573) -> (all lower case string=w574:string)
                n267 = To Lower Case(string=w576) -> (all lower case string=w572:string)
                n268 = To Lower Case(string=w577) -> (all lower case string=w579:string)
                n269 = Match Pattern(string=w572, regular expression=w574) -> (offset past match=w575:i32)  [unwired: 1 in, 3 out]
                n270 = Match Pattern(string=w572, regular expression=w579) -> (offset past match=w578:i32)  [unwired: 1 in, 3 out]
                n271 = Less Than 0?(x=w575) -> (x < 0?=w571:bool)
                n272 = Greater Or Equal To 0?(x=w578) -> (x >= 0?=w570:bool)
                n273 = And(x=w571, y=w570) -> (x .and. y?=w569:bool)
                n274 = case shown="True" w569 {
                  tunnel: w576 -> [_ w597]
                  tunnel: w584 -> [_ w596]
                  tunnel: w583 -> [w586 w594]
                  tunnel: [w586 w593] -> w582
                  tunnel: w581 -> [w585 w591]
                  tunnel: [w585 w591] -> w580
                  tunnel: w568 -> [_ w588]
                  frame False {
                  }
                  frame True {
                    w590 = ""
                    n275 = Build Path(base path=w596, name or relative path=w597) -> (appended path=w595:path)
                    n276 = Path To String(path=w595) -> (string=w587:string)
                    n277 = Search/Split String(string=w587, offset (0)=w588) -> (match + rest of string=w589:string)  [unwired: 1 in, 2 out]
                    n278 = Build Array(w589, w590, w590, w590, w590, w590, w590) -> (w592:string[])
                    n279 = Build Array (concatenate)(w594, w592) -> (w593:string[][])
                  }
                }
              }
            }
          }
        }
        n280 = Array Size(array=w491) -> (size(s)=w490:i32[])
        n281 = property on="file list" class="MCListbox (strict)"("Item Names"=w491, "Disabled"=w486) -> ()  [unwired: 2 in, 2 out]
        n282 = case shown="Error" w481 {
          selector: w481 -> [_ w502]
          frame No Error {
          }
          frame Error {
            n283 = Unbundle(w502) -> ("code"=w500:i32, "source"=w499:string)  [unwired: 1 out]
            n284 = Format Into String(format string="Error with code %d at %s", w500, w499) -> (resulting string=w498:string)  [unwired: 2 in, 1 out]
            n285 = One Button Dialog(message=w498) -> ()  [unwired: 1 in, 1 out]
          }
        }
        n286 = Index Array(array=w490, index=0) -> (element=w488:i32)
        n287 = Build Array (concatenate)(w497, w482) -> (w492:T1[])
        n288 = Initialize Array(refnum<vi> refnum ("vi reference"), w488) -> (w489:refnum<vi>[])
      }
      frame "cleanup" {
        w600 = u8 0 items=["enabled", "disabled", "grayed"] ("disabled state")
        w601 = T1[] [enum."stop"] items=["empty queue", "adjust size", "load", "ld open", "ld calls", "ld system&exec", "unload", "unload templates", "open selected", "update stats", "ablement", "initialize", "cleanup", "stop"] ("Array Constant")
        n289 = property on="file list" class="MCListbox (strict)"("Item Names"=string[][] []) -> ()  [unwired: 2 in, 2 out]
        n290 = property on="file list" class="MCListbox (strict)"("Disabled"=w600) -> ()  [unwired: 2 in, 2 out]
        n291 = property on="stop" class="Bool"("Disabled"=w600) -> ()  [unwired: 2 in, 2 out]
        n292 = property on="reinitialize" class="Bool"("Disabled"=w600) -> ()  [unwired: 2 in, 2 out]
        n293 = property on="load selected" class="Bool"("Disabled"=w600) -> ()  [unwired: 2 in, 2 out]
        n294 = property on="load all" class="Bool"("Disabled"=w600) -> ()  [unwired: 2 in, 2 out]
        n295 = property on="open selected" class="Bool"("Disabled"=w600) -> ()  [unwired: 2 in, 2 out]
      }
      frame "stop" {
        n296 = invoke class="VI" method="FP.Close"() -> ()  [unwired: 3 in, 3 out]
      }
    }
  }
